vi "Canbus frame to LEIN.vi"(1 "Data Length":u32, 2 "IsRemote(0)":u8, 5 "Data":u8[](array[numeric]), 11 "error in (no error)":errorcluster, 12 "ArbitrationID":u32) -> (8 "CMD":T1={"SID"=0, "ANF"=FALSE, "CMD"=enum."TASK", "DATA"=[]}, 10 "LEIN Frame":bool, 15 "error out":errorcluster)   [LabVIEW 2010]
uses:
  Defenitions/LEIN CMD Cluster.ctl
  Defenitions/LEIN CMD List.ctl
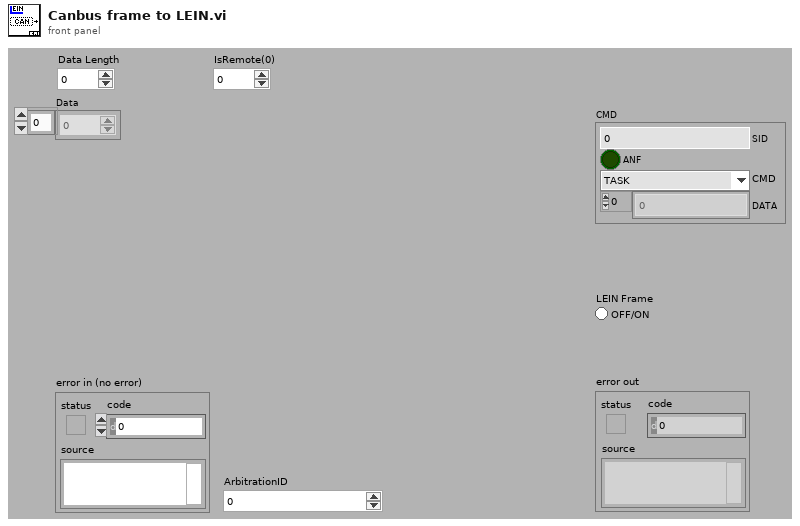
[diagram p1: front panel]
types:
  T1 = typedef "LEIN CMD Cluster.ctl" = cluster{"SID":u8, "ANF":bool, "CMD":T2, "DATA":u8[]}
  T2 = typedef "LEIN CMD List.ctl" = enum8{"ACTI", "TASK", "RES0", "STAT", "RES1", "RES2", "RES3", "USER"}
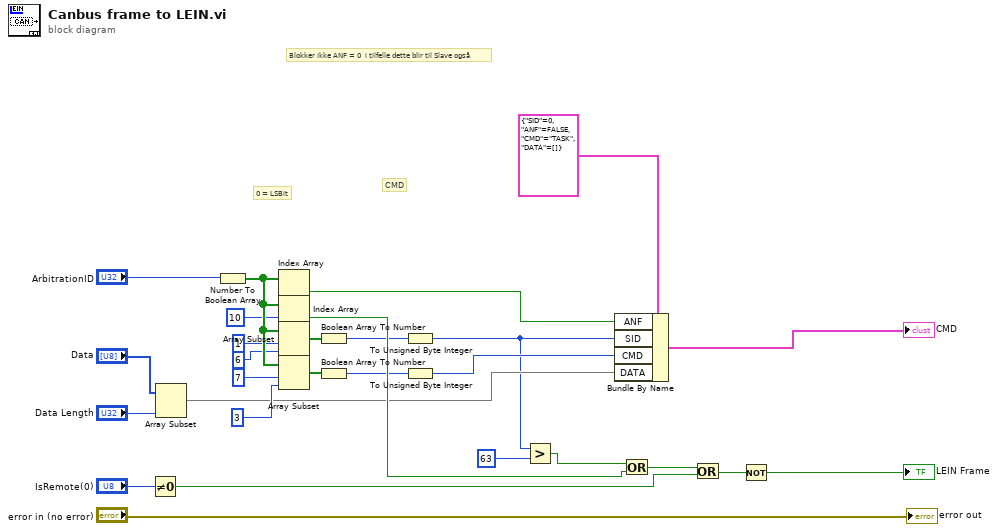
[diagram p0: block diagram]
diagram:
  # "CMD"
  # "0 = LSBit"
  # "Blokker ikke ANF = 0  i tilfelle dette blir til Slave også"
  n1 = Not Equal To 0?(x="IsRemote(0)") -> (x != 0?=w4:bool)
  n2 = Array Subset(array="Data", length="Data Length") -> (w7:u8[])  [unwired: 1 in]
  n3 = Number To Boolean Array(number="ArbitrationID") -> (Boolean array=w22:bool[])
  n4 = Index Array(array=w22) -> (element=w23:bool)  [unwired: 1 in]
  n5 = Index Array(array=w22, index=10) -> (element=w25:bool)
  n6 = Array Subset(array=w22, index=1, length=6) -> (w16:bool[])
  n7 = Array Subset(array=w22, index=7, length=3) -> (w17:bool[])
  n8 = Boolean Array To Number(Boolean array=w16) -> (number=w19:u32)
  n9 = Boolean Array To Number(Boolean array=w17) -> (number=w20:u32)
  n10 = To Unsigned Byte Integer(number=w19) -> (unsigned 8bit integer=w2:u8)
  n11 = To Unsigned Byte Integer(number=w20) -> (unsigned 8bit integer=w21:u8)
  n12 = Greater?(x=w2, y=u8 63) -> (0:w1:bool)
  n13 = Bundle By Name(cluster=T1 {"SID"=0, "ANF"=FALSE, "CMD"=enum."TASK", "DATA"=[]} ("CMD"), "ANF"=w23, "SID"=w2, "CMD"=w21, "DATA"=w7) -> (→"CMD":T1)
  n14 = Or(x=w1, y=w25) -> (x .or. y?=w26:bool)
  n15 = Or(x=w26, y=w4) -> (x .or. y?=w6:bool)
  n16 = Not(x=w6) -> (.not. x?=→"LEIN Frame":bool)
  "error out" <- "error in (no error)"
